vi "newport_testing.vi"() -> ()   [LabVIEW 2017]
uses:
  Newport ESP301/Newport ESP301.lvlib
panel:
  out "error out 3":errorcluster
  in  "error in (no error) 3":errorcluster
  in  "Wait before read (0ms)":u32
  in  "Bytes to read (100)":u32=100
  out "Returned string":string
  in  "Command":string
  out "error out 2":errorcluster={"status"=TRUE, "code"=-1073807339, "source"="VISA Read dans Newport ESP301.lvlib:Write Command and Read.vi"}
  in  "error in (no error) 2":errorcluster
  in  "Serial Link (RS232)":enum16{"RS232", "USB"}(ring)
  out "error out":errorcluster {"code" format="%.0x"}
  in  "VISA resource name":refnum<visa-resource-name>
  in  "error in (no error)":errorcluster
  in  "ID Query (True)":bool=TRUE
  in  "Reset (False)":bool
  # "INITIALIZATION"
  # "(c) 2009 <Newport>.  ALL RIGHTS RESERVED."
  # "WRITE COMMAND AND READ"
  # "CLOSE"
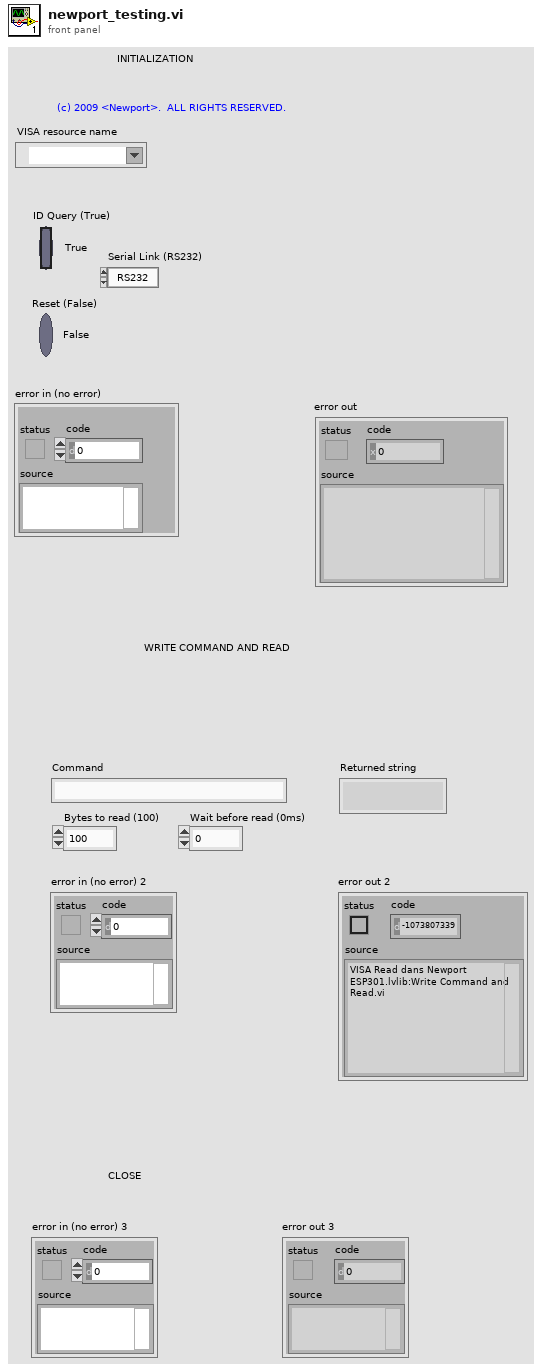
[diagram p1: front panel]
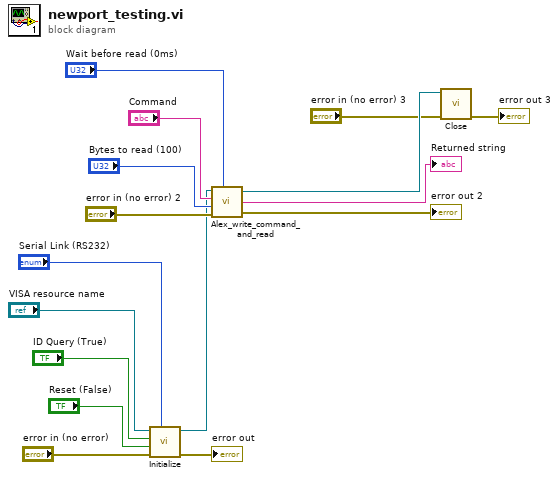
[diagram p0: block diagram]
diagram:
  n1 = call "Initialize.vi"("VISA resource name"="VISA resource name", "ID Query (True)"="ID Query (True)", "Reset (False)"="Reset (False)", "error in (no error)"="error in (no error)", "Serial Link (RS232)"="Serial Link (RS232)") -> ("VISA resource name out"=w4:refnum<visa-resource-name>, "error out"=→"error out":errorcluster)  [unwired: 4 in]
  n2 = call "Alex_write_command_and_read.vi"("VISA resource name"=w4, "Wait before read (0ms)"="Wait before read (0ms)", "Command"="Command", "Bytes to read (100)"="Bytes to read (100)", "error in (no error)"="error in (no error) 2") -> ("VISA resource name out"=w3:refnum<visa-resource-name>, "Returned string"=→"Returned string":string, "error out"=→"error out 2":errorcluster)  [unwired: 1 in]
  n3 = call "Close.vi"("error in (no error)"="error in (no error) 3", "VISA resource name"=w3) -> ("error out"=→"error out 3":errorcluster)  [unwired: 9 in]
